vi "Video Stuff v06.vi"() -> ()   [LabVIEW 2009]
uses:
  <vilib>/vision/NI_Vision_Development_Module.lvlib
  <vilib>/vision/driver/NI_Vision_Acquisition_Software.lvlib
  <vilib>/Instr/_visa.llb/VISA Configure Serial Port (Instr).vi
  <vilib>/userDefined/High Color/IMAQdx.ctl
panel:
  in  "VISA resource name":refnum<visa-resource-name>
  out "Occupancy Grid Square Size":dbl
  in  "LIDAR/Wheel Position Offset (in.)":dbl=30.0
  out "\"Obstickles\" y":dbl[](array[numeric])
  out "\"Obstickles\" x":dbl[](array[numeric])
  in  "Max Width of Vision (in.)":i32=84
  out "Small":T1(plugin-control)
  in  "Resolution of Small Image":i32=36
  out "Super Filter":T1(plugin-control)
  in  "Color Mode":u16(ring) items=["RGB", "HSL", "HSV", "HSI"]
  in  "Blue Range":cluster{"Lower value":i32, "Upper value":i32}={"Lower value"=250, "Upper value"=255}
  in  "Green Range":cluster{"Lower value":i32, "Upper value":i32}={"Lower value"=250, "Upper value"=255}
  in  "Red Range":cluster{"Lower value":i32, "Upper value":i32}={"Lower value"=240, "Upper value"=255}
  in  "stop":bool
  out "trans":T1(plugin-control)
  out "Buffer Number":u32
  out "Live Video":T1(plugin-control)
  in  "Video Modes":i32(listbox)=20
  in  "Camera Name":T2="cam0"
  in  "Calibration File Path":path=path "C:/Users/Nick/Desktop/eric/calibrationGrid.PNG"
  out "Top Image":T1(plugin-control) caption="Calibration Template"
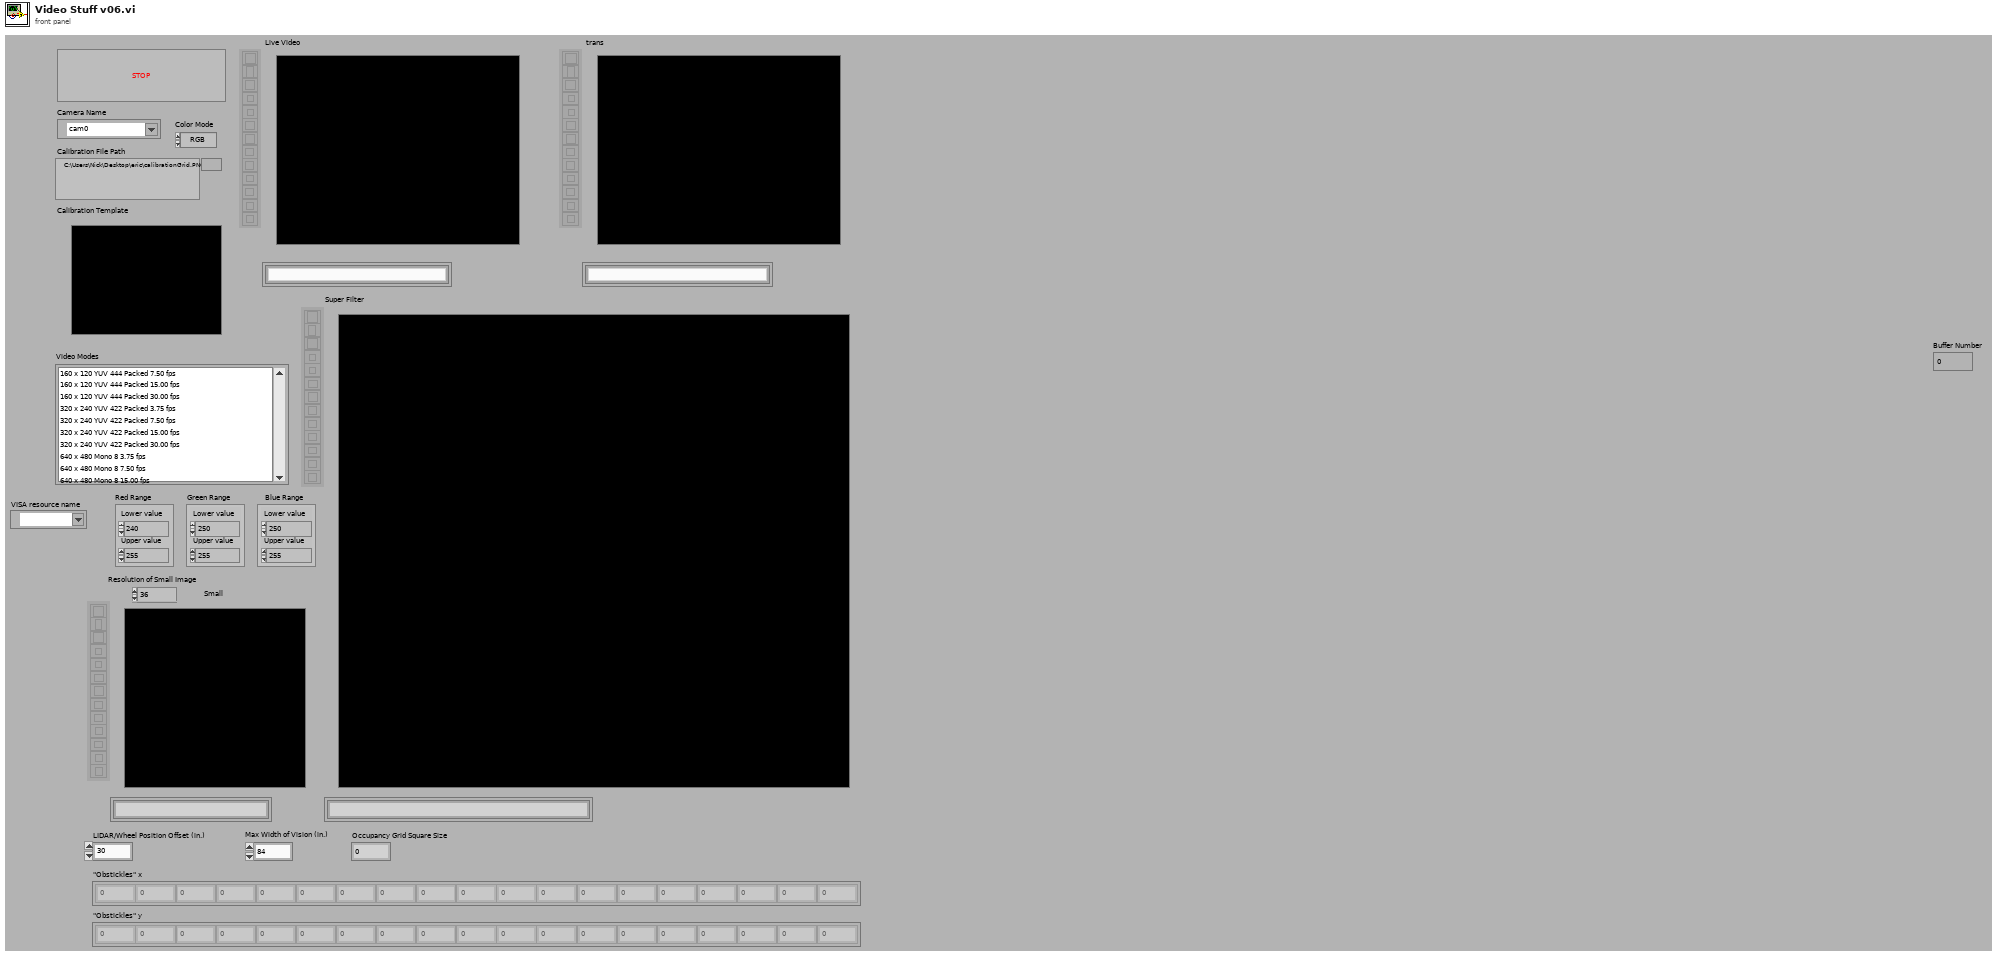
[diagram p1: front panel]
types:
  T1 = typedef "IMAQ Image.ctl" = refnum<image>
  T2 = typedef "IMAQdx.ctl" = refnum<k21>
  T3 = typedef "Image Type" = u32
  T4 = cluster{"X Step":sgl, "Y Step":sgl, "Unit":u32, "Threshold Range":cluster{"Lower value":sgl, "Upper value":sgl}}
  T5 = cluster{"Distortion":u32, "Corrected Image Scaling":u32, "Corrected Image Learn ROI":u32, "Learn Error Map?":bool, "Learn Correction Table?":bool}
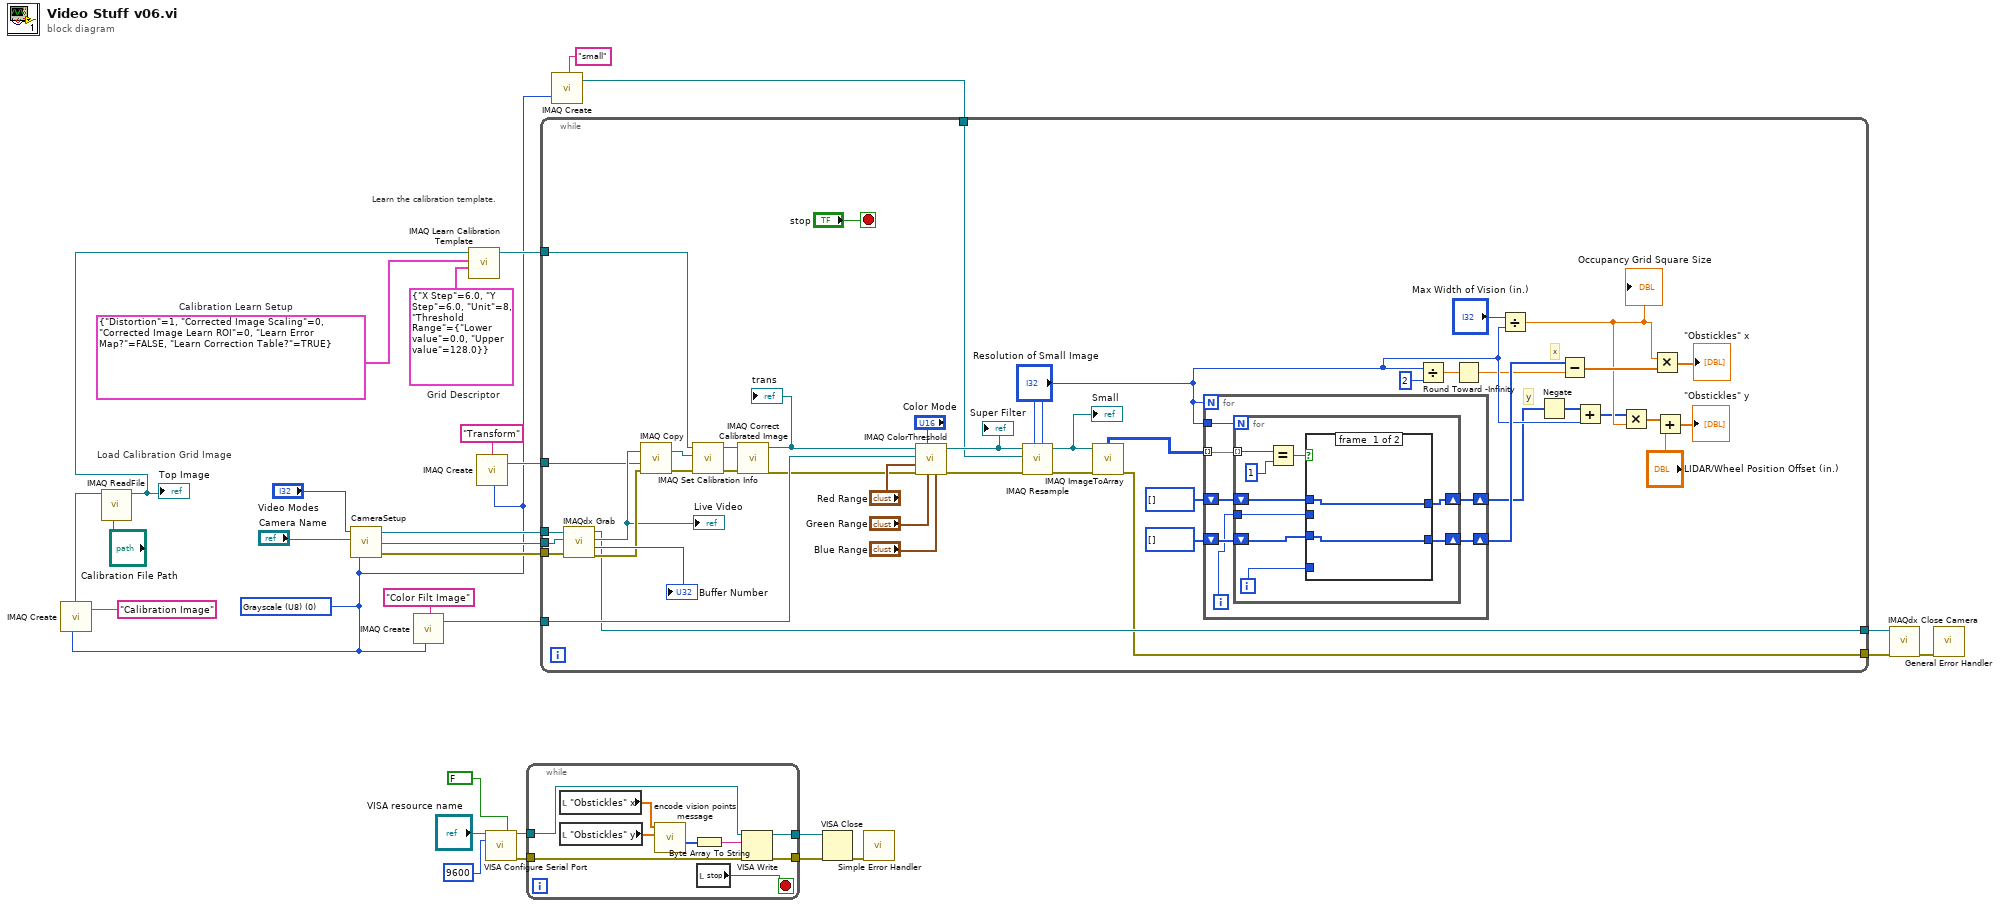
[diagram p0: block diagram]
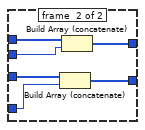
[diagram p2: hidden frame]
diagram:
  w13 = T3 0 items=["Grayscale (U8)", "Grayscale (I16)", "Grayscale (SGL)", "Complex (CSG)", "RGB (U32)", "HSL (U32)", "RGB (U64)", "Grayscale (U16)"] ("Image Type")
  w29 = T4 {"X Step"=6.0, "Y Step"=6.0, "Unit"=8, "Threshold Range"={"Lower value"=0.0, "Upper value"=128.0}}  # Grid Descriptor
  w30 = T5 {"Distortion"=1, "Corrected Image Scaling"=0, "Corrected Image Learn ROI"=0, "Learn Error Map?"=FALSE, "Learn Correction Table?"=TRUE}  # Calibration Learn Setup
  # "Load Calibration Grid Image"
  # "Learn the calibration template."
  n1 = call "IMAQ Create"("Image Name"="Calibration Image", "Image Type"=w13) -> ("New Image"=w17:T1)  [unwired: 2 in, 2 out]
  n2 = call "IMAQ ReadFile"("File Path"="Calibration File Path", "Image"=w17) -> ("Image Out"=w16:T1)  [unwired: 3 in, 6 out]
  "Top Image" <- w16
  n3 = call "CameraSetup.vi"("Image Type"=w13, "Camera Name"="Camera Name", "Video Modes"="Video Modes") -> ("error out"=w18:errorcluster, "New Image"=w19:T1, "Session Out"=w20:T2)  [unwired: 1 in]
  n4 = call "IMAQ Create"("Image Name"="Color Filt Image", "Image Type"=w13) -> ("New Image"=w15:T1)  [unwired: 2 in, 2 out]
  n5 = call "IMAQ Learn Calibration Template"("Grid Descriptor"=w29, "Calibration Learn Setup"=w30, "Image"=w16) -> ("Calibrated Image"=w22:T1)  [unwired: 4 in, 4 out]
  n6 = call "IMAQ Create"("Image Name"="Transform", "Image Type"=w13) -> ("New Image"=w21:T1)  [unwired: 2 in, 2 out]
  n7 = call-poly "VISA Configure Serial Port"("VISA resource name"="VISA resource name", "Enable Termination\nChar (T)"=FALSE ("Enable Termination\nChar (T)"), "baud rate (9600)"=u32 9600) -> ("VISA resource name out"=w4:refnum<visa-resource-name>, "error out"=w1:errorcluster)  [unwired: 11 in]
  n8 = while {
    tunnel: w4 -> [w35]
    tunnel: [w34] -> w8
    tunnel: [w33] -> w6
    tunnel: w1 -> [w31]
    stop <- w32 stop-if-true
    n9 = local read "\"Obstickles\" x"() -> (w39:dbl[])
    n10 = local read "\"Obstickles\" y"() -> (w38:dbl[])
    n11 = call "encode vision points message.vi"("y locations"=w38, "x locations"=w39) -> ("vision points message"=w37:u8[])  [unwired: 9 in]
    n12 = Byte Array To String(unsigned byte array=w37) -> (string=w36:string)
    n13 = local read "stop"() -> (w32:bool)
    n14 = VISA Write(VISA resource name=w35, write buffer=w36, error in (no error)=w31) -> (VISA resource name out=w34:refnum<visa-resource-name>, error out=w33:errorcluster)  [unwired: 1 out]
  }
  n15 = call "IMAQ Create"("Image Name"="small", "Image Type"=w13) -> ("New Image"=w12:T1)  [unwired: 2 in, 2 out]
  n16 = while {
    tunnel: w22 -> [w77]
    tunnel: w21 -> [w76]
    tunnel: w20 -> [w75]
    tunnel: w19 -> [w74]
    tunnel: w18 -> [w73]
    tunnel: w15 -> [w62]
    tunnel: w12 -> [w60]
    tunnel: [w58] -> w10
    tunnel: [w57] -> w9
    stop <- "stop" stop-if-true
    # "y"
    # "x"
    n17 = call <vilib>:"IMAQdx Grab.vi"("error in"=w73, "Image In"=w74, "Session In"=w75) -> ("error out"=w79:errorcluster, "Buffer Number Out"=→"Buffer Number":u32, "Image Out"=w78:T1, "Session Out"=w58:T2)  [unwired: 1 in, 4 out]
    "Live Video" <- w78
    n18 = call "IMAQ Copy"("error in (no error)"=w79, "Image Dst"=w76, "Image Src"=w78) -> ("error out"=w80:errorcluster, "Image Dst Out"=w83:T1)  [unwired: 3 in]
    n19 = call "IMAQ Set Calibration Info"("error in (no error)"=w80, "Image Dst"=w83, "Image Src"=w77) -> ("error out"=w81:errorcluster, "Calibrated Image"=w82:T1)  [unwired: 1 in, 6 out]
    n20 = call "IMAQ Correct Calibrated Image"("error in (no error)"=w81, "Image Src"=w82) -> ("error out"=w61:errorcluster, "Corrected Image"=w63:T1)  [unwired: 5 in, 3 out]
    "trans" <- w63
    n21 = call "IMAQ ColorThreshold"("Blue or Luma or Val or Inten Range"="Blue Range", "Green or Sat Range"="Green Range", "Color Mode"="Color Mode", "error in (no error)"=w61, "Red or Hue Range"="Red Range", "Image Dst"=w62, "Image Src"=w63) -> ("error out"=w68:errorcluster, "Image Dst Out"=w67:T1)  [unwired: 3 in]
    "Super Filter" <- w67
    n22 = call "IMAQ Resample"("X Resolution"="Resolution of Small Image", "Y Resolution"="Resolution of Small Image", "error in (no error)"=w68, "Image Dst"=w60, "Image Src"=w67) -> ("error out"=w66:errorcluster, "Image Dst Out"=w65:T1)  [unwired: 5 in]
    "Small" <- w65
    n23 = call "IMAQ ImageToArray"("error in (no error)"=w66, "Image"=w65) -> ("error out"=w57:errorcluster, "Image Pixels (U8)"=w54:u8[][])  [unwired: 2 in, 3 out]
    n24 = for {
      N: "Resolution of Small Image" -> [_]
      tunnel: "Resolution of Small Image" -> [w91]
      tunnel: w54 -> [w90] mode=indexing
      shift-right: [w89] -> w53
      shift-left: i32[] [] -> [w88]
      shift-right: [w86] -> w42
      shift-left: i32[] [] -> [w85]
      i -> [w87]
      n25 = for {
        N: w91 -> [_]
        tunnel: w90 -> [w100] mode=indexing
        shift-right: [w96] -> w89
        shift-left: w88 -> [w95]
        tunnel: w87 -> [w94]
        shift-right: [w93] -> w86
        shift-left: w85 -> [w92]
        i -> [w98]
        n26 = Equal?(x=w100, y=u8 1) -> (x = y?=w97:bool)
        n27 = case shown="False" w97 {
          tunnel: w98 -> [_ w108]
          tunnel: [w101 w107] -> w96
          tunnel: w95 -> [w101 w106]
          tunnel: w94 -> [_ w105]
          tunnel: [w102 w104] -> w93
          tunnel: w92 -> [w102 w103]
          frame #0 {
          }
          frame #1 {
            n28 = Build Array (concatenate)(w106, w108) -> (w107:i32[])
            n29 = Build Array (concatenate)(w103, w105) -> (w104:i32[])
          }
        }
      }
    }
    n30 = Divide(x="Resolution of Small Image", y=2) -> (x/y=w41:dbl)
    n31 = Round Toward -Infinity(1:w41) -> (0:w40:dbl)
    n32 = Divide(x="Max Width of Vision (in.)", y="Resolution of Small Image") -> (x/y=w48:dbl)
    "Occupancy Grid Square Size" <- w48
    n33 = Negate(x=w42) -> (-x=w43:i32[])
    n34 = Subtract(x=w53, y=w40) -> (x-y=w49:dbl[])
    n35 = Add(x=w43, y="Resolution of Small Image") -> (x+y=w47:i32[])
    n36 = Multiply(x=w47, y=w48) -> (x*y=w44:dbl[])
    n37 = Multiply(x=w48, y=w49) -> (x*y=→"\"Obstickles\" x":dbl[])
    n38 = Add(x=w44, y="LIDAR/Wheel Position Offset (in.)") -> (x+y=→"\"Obstickles\" y":dbl[])
  }
  n39 = VISA Close(VISA resource name=w8, error in (no error)=w6) -> (error out=w7:errorcluster)
  n40 = call <vilib>:"Simple Error Handler.vi"("error in (no error)"=w7) -> ()  [unwired: 4 in, 5 out]
  n41 = call <vilib>:"IMAQdx Close Camera.vi"("error in"=w9, "Session In"=w10) -> ("error out"=w11:errorcluster)  [unwired: 9 out]
  n42 = call <vilib>:"General Error Handler.vi"("error in (no error)"=w11) -> ()  [unwired: 1 in, 14 out]
